vi "SetClearingMode.vi"(9 "Clear mode":refnum<vi>, 10 "Clearing modes":refnum<vi>, 11 ".NET Refnum in":refnum<k24>) -> ()   [LabVIEW 2019]
uses:
  Dependencies/PVCamNET.dll
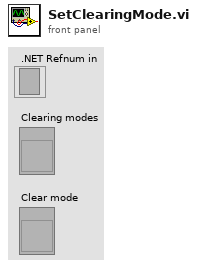
[diagram p1: front panel]
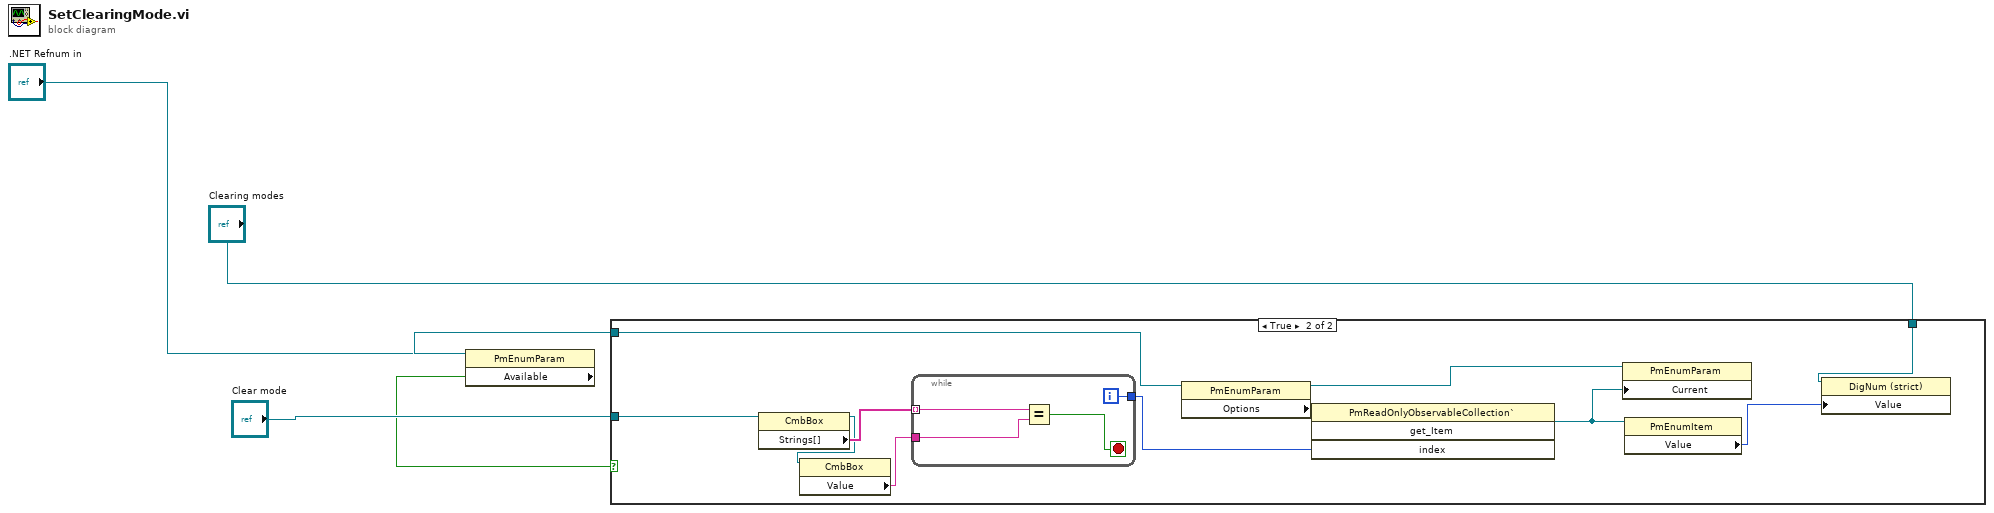
[diagram p0: block diagram]
diagram:
  n1 = property class="PmEnumParam"(reference=".NET Refnum in") -> (reference out=w3:refnum<k24>, "Available"=w2:bool)  [unwired: 1 in, 1 out]
  n2 = case shown="True" w2 {
    tunnel: w3 -> [_ w15]
    tunnel: "Clearing modes" -> [_ w10]
    tunnel: "Clear mode" -> [_ w8]
    frame False {
    }
    frame True {
      n3 = property class="CmbBox"(reference=w8) -> (reference out=w7:refnum<vi>, "Strings[]"=w16:string[])  [unwired: 1 in, 1 out]
      n4 = property class="CmbBox"(reference=w7) -> ("Value"=w6:string)  [unwired: 1 in, 2 out]
      n5 = while {
        tunnel: w16 -> [w20] mode=indexing
        tunnel: [w18] -> w13
        tunnel: w6 -> [w17]
        i -> [w18]
        stop <- w19 stop-if-true
        n6 = Equal?(x=w20, y=w17) -> (x = y?=w19:bool)
      }
      n7 = property class="PmEnumParam"(reference=w15) -> (reference out=w11:refnum<k24>, "Options"=w14:refnum<k24>)  [unwired: 1 in, 1 out]
      n8 = invoke class="PmReadOnlyObservableCollection`" method="get_Item"(reference=w14, "index"=w13) -> ("get_Item"=w12:refnum<k24>)  [unwired: 2 in, 3 out]
      n9 = property class="PmEnumParam"(reference=w11, "Current"=w12) -> ()  [unwired: 1 in, 2 out]
      n10 = property class="PmEnumItem"(reference=w12) -> ("Value"=w9:i32)  [unwired: 1 in, 2 out]
      n11 = property class="DigNum (strict)"(reference=w10, "Value"=w9) -> ()  [unwired: 1 in, 2 out]
    }
  }
